vi "SECoP-createNode_2.vi"(6 "Interface":string="127.0.0.1", 7 "description":string, 8 "error in (no error)":errorcluster, 9 "TCP port":u16=2055, 10 "node id":string, 11 "DLL path (in)":T1) -> (0 "error out":errorcluster, 3 "DLL path (out)":T1)   [LabVIEW 2023, in "SECoP.lvlib"]
doc: "Call <b>\"SECoP-createNode2.vi\"</b> to create an empty SECoP node and bind it to a specific interface and port. You need at least one for a working SEC-node. Every node exists independent of each other, but it is up to the user, how they act.\n\n<b>DLL path</b> input and output of cluster from \"SECoP-Initialize.vi\"\n<b>node id</b> unique name of the SECoP node\n<b>description</b> a mandatory description text\n<b>Interface</b> IP address of interface to bind to (0.0.0.0 or :: for any interface)\n<b>TCP port</b> port to listen to"
uses:
  SECoP.lvlib
  SECoP-libraries.ctl
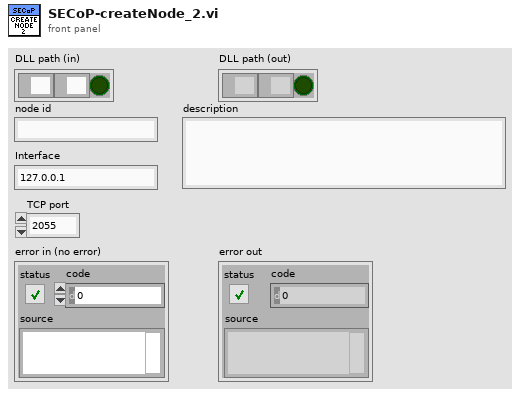
[diagram p1: front panel]
types:
  T1 = typedef "SECoP.lvlib/SECoP-libraries.ctl" = cluster{"serverDLL":path, "variantDLL":path, "cleanup_mode":bool}
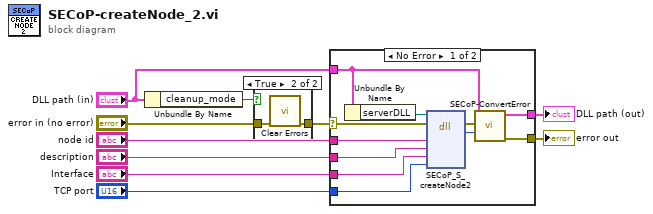
[diagram p0: block diagram]
diagram:
  n1 = Unbundle By Name("DLL path (in)") -> ("cleanup_mode"=w5:bool)
  n2 = case shown="True" w5 {
    tunnel: "error in (no error)" -> [w11 w13]
    tunnel: [w11 w12] -> w3
    frame False {
    }
    frame True {
      n3 = call <vilib>:"Clear Errors.vi"("error in (no error)"=w13) -> ("error out"=w12:errorcluster)  [unwired: 5 in, 1 out]
    }
  }
  n4 = case shown="No Error" w3 {
    selector: w3 -> [w22 w25]
    tunnel: "DLL path (in)" -> [w14 w26]
    tunnel: [w23 w26] -> w10
    tunnel: [w24 w25] -> w9
    tunnel: "node id" -> [w19 _]
    tunnel: "description" -> [w18 _]
    tunnel: "TCP port" -> [w17 _]
    tunnel: "Interface" -> [w16 _]
    frame No Error {
      n5 = Unbundle By Name(w14) -> ("serverDLL"=w15:path)
      n6 = dll-call lib="Z:/Praktische_Aufgaben/SECoP-LabVIEW2015/32bit/SECoP32.dll" fn="SECoP_S_createNode2"(path in=w15, error in=w22, "id"=w19, "description"=w18, "interface"=w16, "TCP port"=w17) -> (error out=w21:errorcluster, "return type"=w20:i32)  [unwired: 5 in, 1 out]
      n7 = call "SECoP-ConvertError.vi"("return code"=w20, "error in (no error)"=w21, "DLL path (in)"=w14) -> ("error out"=w24:errorcluster, "DLL path (out)"=w23:T1)  [unwired: 7 in]
    }
    frame Error {
    }
  }
  "DLL path (out)" <- w10
  "error out" <- w9
